vi "Set Initialization Data - Settings View.vi"(8 "error in":errorcluster, 11 "Main View in":refnum<class "Main View.lvclass">) -> (0 "error out":errorcluster, 3 "Main View out":refnum<class "Main View.lvclass">)   [LabVIEW 2018, in "Main View.lvclass"]
doc: "Sets the initialization data of a statically linked subWorker."
uses:
  Main View.lvclass
  Settings View/Initialization Data.ctl
  Main View.lvclass/Main View.ctl
  Settings View/Settings View.lvclass
  D:/Program Files (x86)/National Instruments/LabVIEW 2018/vi.lib/addons/_Workers/Library/Classes/Worker/Worker.lvclass
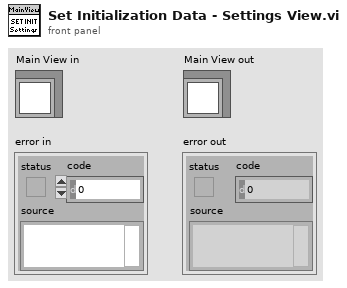
[diagram p1: front panel]
types:
  T1 = typedef "Settings View.lvclass/Initialization Data.ctl" = cluster{"MainPanel":refnum<vi>}
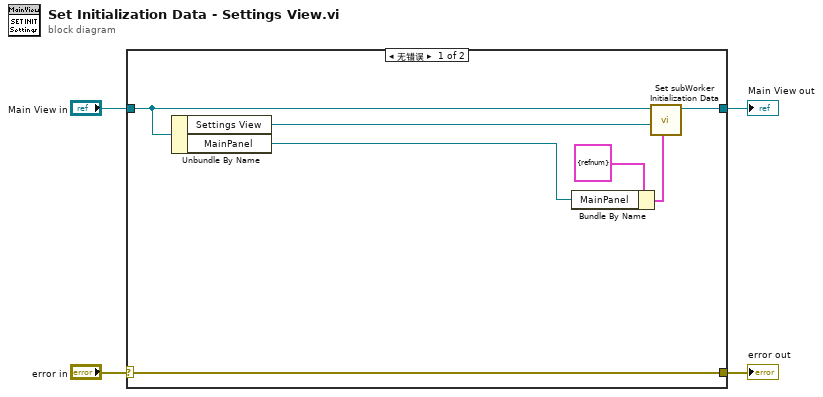
[diagram p0: block diagram]
diagram:
  n1 = case shown="无错误" "error in" {
    selector: "error in" -> [w11 w13]
    tunnel: [w11 w13] -> w3
    tunnel: [w9 w12] -> w2
    tunnel: "Main View in" -> [w8 w12]
    frame No Error {
      n2 = Unbundle By Name(w8) -> ("Settings View"=w10:refnum<class "Settings View.lvclass">, "MainPanel"=w5:refnum<vi>)
      n3 = Bundle By Name(cluster=T1 {"MainPanel"=refnum} ("Initialization Data"), "MainPanel"=w5) -> (w6:T1)
      n4 = call-dynamic "Set subWorker Initialization Data.vi"("Initialization Data"=w6, "subWorker"=w10, "Worker"=w8) -> ("Worker out"=w9:refnum<class "Main View.lvclass">)  [unwired: 8 in]
    }
    frame Error {
    }
  }
  "error out" <- w3
  "Main View out" <- w2
